vi "New Default Trigger.vi"(8 "error in (no error)":errorcluster, 11 "Default State":bool) -> (0 "error out":errorcluster, 3 "Default Trigger out":refnum<class "Default Trigger.lvclass">)   [LabVIEW 2015, in "Waveform Data Logger Engine.lvlib" / "Default Trigger.lvclass"]
uses:
  Default Trigger.lvclass
  Default Trigger.lvclass/Default Trigger.ctl
  Trigger/Trigger Type.ctl
  Trigger/Trigger.lvclass/Trigger.ctl
  Trigger/Write Trigger Type.vi
  Trigger/Trigger.lvclass
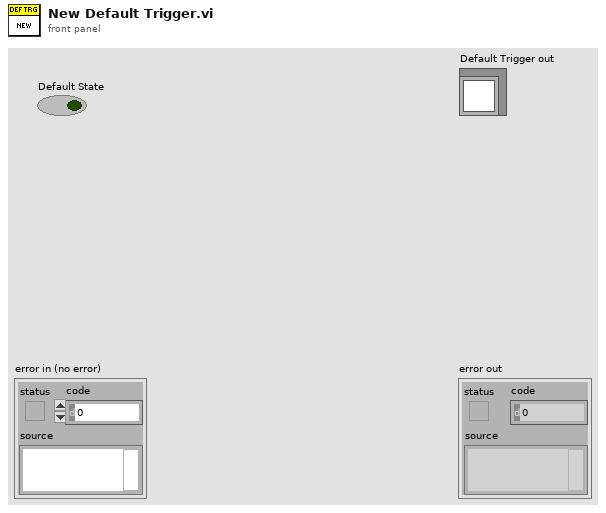
[diagram p1: front panel]
types:
  T1 = typedef "Waveform Data Logger Engine.lvlib/Trigger.lvclass/Trigger Type.ctl" = enum16{"Default", "Digital Edge", "Analog Edge", "In Range", "Value Change", "Boolean Evaluation"}
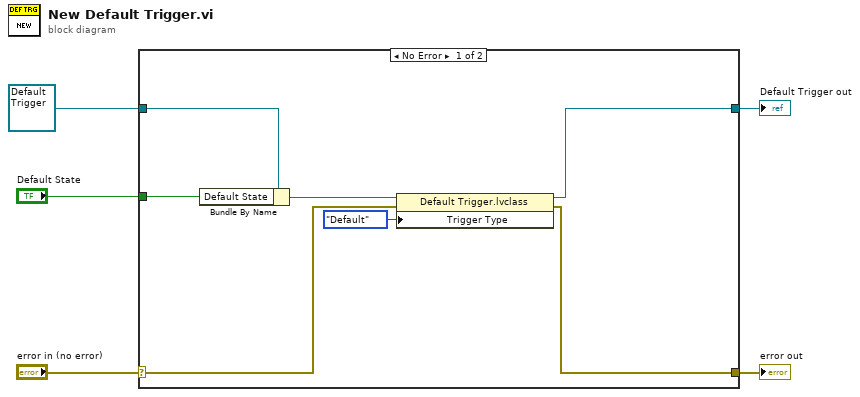
[diagram p0: block diagram]
diagram:
  n1 = case shown="No Error" "error in (no error)" {
    selector: "error in (no error)" -> [w9 w14]
    tunnel: [w8 w14] -> w4
    tunnel: [w7 w13] -> w2
    tunnel: refnum<class "Default Trigger.lvclass"> refnum ("Default Trigger in") -> [w12 w13]
    tunnel: "Default State" -> [w11 _]
    frame No Error {
      n2 = Bundle By Name(cluster=w12, "Default State"=w11) -> (w10:refnum<class "Default Trigger.lvclass">)
      n3 = property class="Default Trigger.lvclass"(reference=w10, error in=w9, "Trigger Type"=Trigger_Type."Default") -> (reference out=w7:refnum<class "Default Trigger.lvclass">, error out=w8:errorcluster)
    }
    frame Error {
    }
  }
  "error out" <- w4
  "Default Trigger out" <- w2
